vi "多参数全局变量.vi"() -> ()   [LabVIEW 2022 SP3, in "斯坦道原位多参数.lvlib"]
uses:
  <vilib>/Plasmionique/MB Master/MB_Master_Serial/MB_Master_Serial.lvclass
panel:
  in  "MB_Serial session in":refnum<class "MB_Master_Serial.lvclass">
  out "pHmv数据区":T1
  out "TDS数据区":T1
  out "spCond数据区":T1
  out "传感器通道号":T2
  out "Sal数据区":T1
  out "NH3N数据区":T1
  out "ORP数据区":T1
  out "蓝绿藻数据区":T1
  out "藻密度数据区":T1
  out "叶绿素数据区":T1
  out "Turb数据区":T1
  out "Cond数据区":T1
  out "DO%数据区":T1
  out "DO数据区":T1
  out "pH数据区":T1
  out "水温数据区":T1
  out "运行状态":string
  out "通讯状态":bool
  out "测量数据区":T3
  out "关键参数区":T4
  in  "控制命令":u16(ring) items=["启动测量"=1, "标样核查"=2, "零点核查"=3, "跨度核查"=4, "空白测试"=5, "平行样测试"=6, "加标回收"=7, "空白校准"=8, "标样校准"=9, "初始化（清洗）"=10, "停止测试"=11, "仪器重启"=12, "校时"=13, "模式设置"=14, "测量间隔设置"=15]
  out "状态告警区":T5
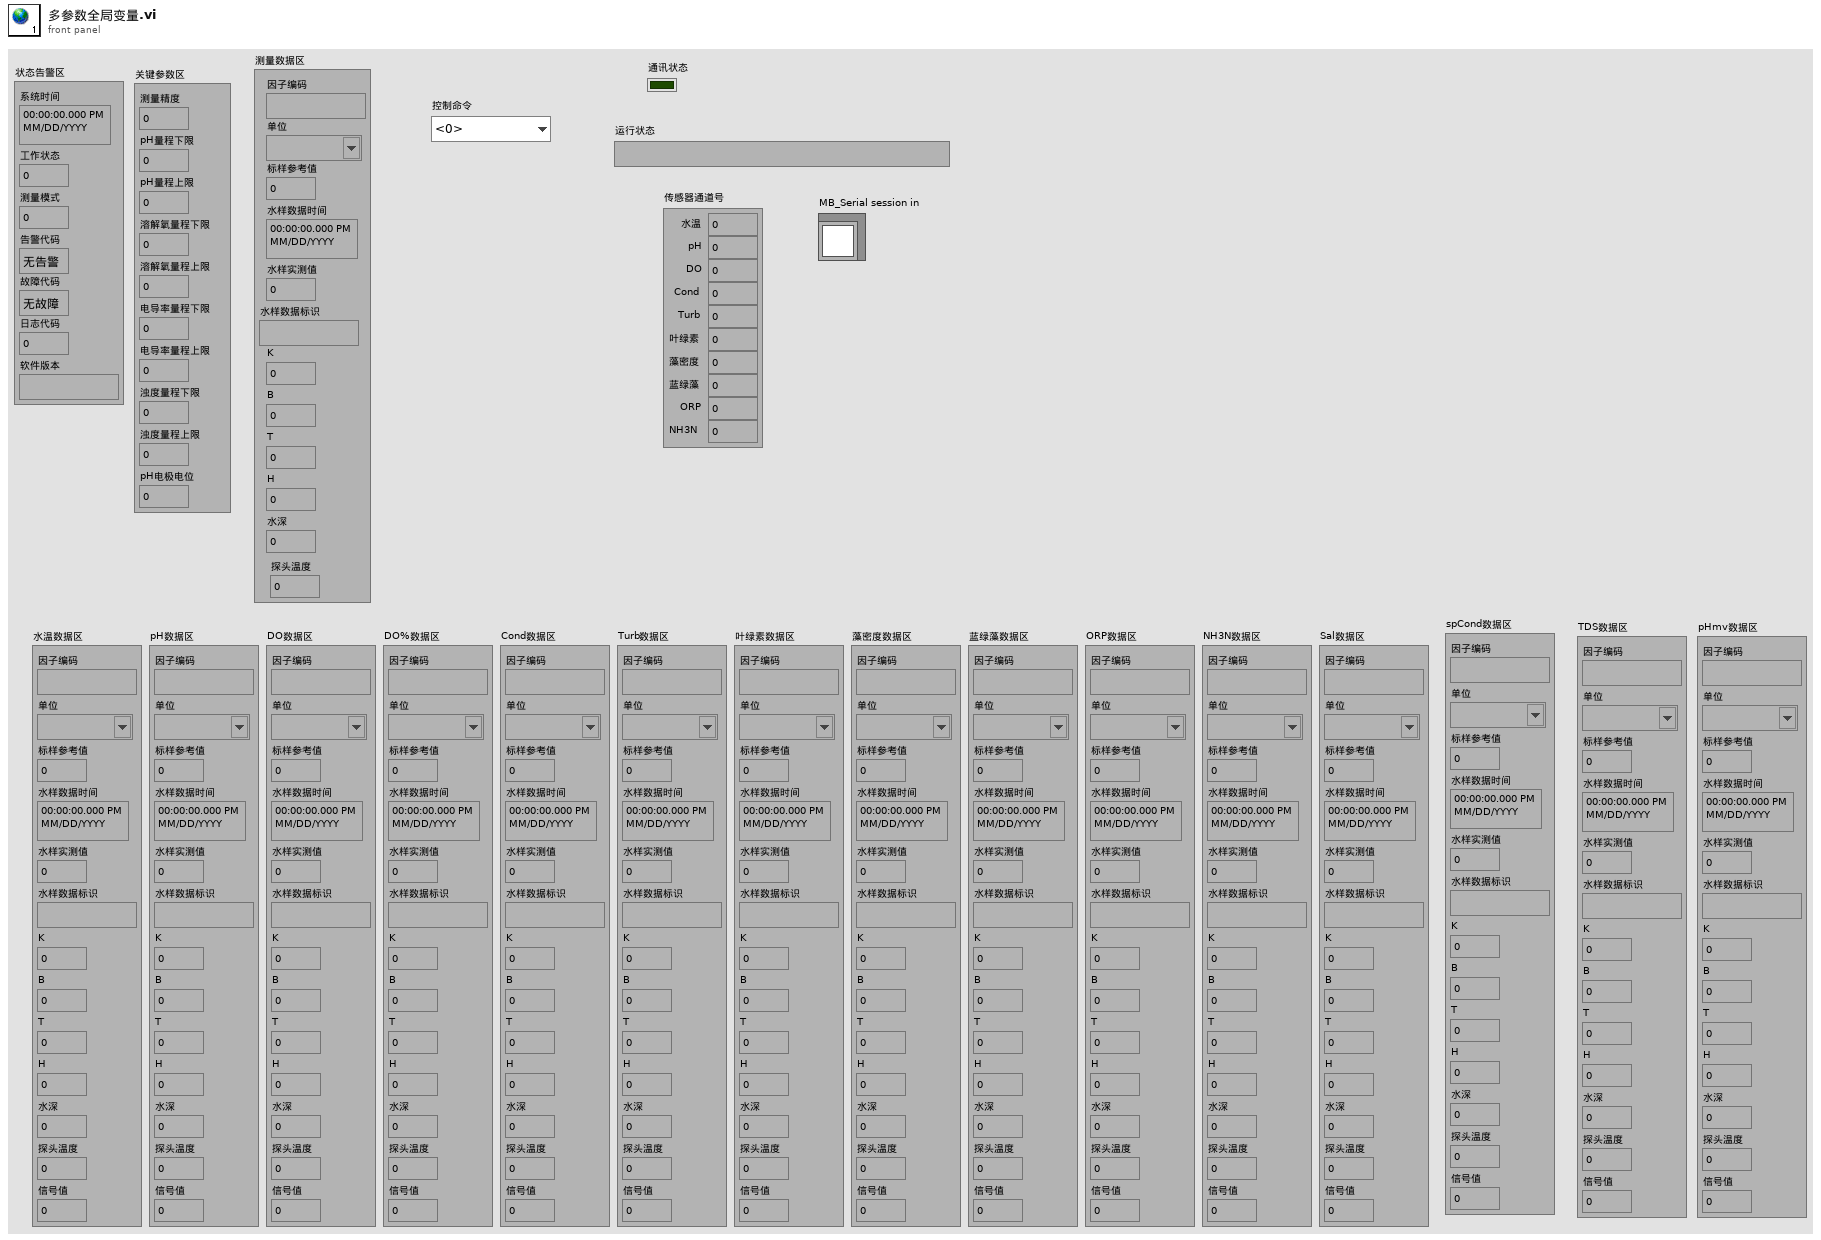
[diagram p1: front panel]
types:
  T1 = cluster{"因子编码":string, "单位":string, "标样参考值":sgl, "水样数据时间":timestamp, "水样实测值":sgl, "水样数据标识":string, "K":sgl, "B":sgl, "T":sgl, "H":sgl, "水深":sgl, "探头温度":sgl, "信号值":sgl}
  T2 = cluster{"水温":dbl, "pH":dbl, "DO":dbl, "Cond":dbl, "Turb":dbl, "叶绿素":dbl, "藻密度":dbl, "蓝绿藻":dbl, "ORP":dbl, "NH3N":dbl}
  T3 = cluster{"因子编码":string, "单位":string, "标样参考值":sgl, "水样数据时间":timestamp, "水样实测值":sgl, "水样数据标识":string, "K":sgl, "B":sgl, "T":sgl, "H":sgl, "水深":sgl, "探头温度":sgl}
  T4 = cluster{"测量精度":u16, "pH量程下限":sgl, "pH量程上限":sgl, "溶解氧量程下限":sgl, "溶解氧量程上限":sgl, "电导率量程下限":sgl, "电导率量程上限":sgl, "浊度量程下限":sgl, "浊度量程上限":sgl, "pH电极电位":sgl}
  T5 = cluster{"系统时间":timestamp, "工作状态":u16, "测量模式":u16, "告警代码":enum16{"无告警", "缺试剂告警", "缺水样告警", "缺蒸馏水告警", "缺标液告警", "仪表漏液告警", "标定异常告警", "超量程告警", "加热异常", "低试剂预警", "超上限告警", "超下限告警", "仪表内部其他异常", "滴定异常告警", "电极异常告警", "量程切换告警", "参数设置告警", "PH电极电位异常", "电导率电极异常", "浊度光度异常", "溶解氧电极异常", "溶解氧光强异常", "温度异常告警", "PH异常告警", "溶解氧异常告警", "电导率异常告警", "浊度异常告警", "叶绿素异常告警", "藻密度异常告警", "蓝绿藻异常告警", "ORP异常告警", "氨氮异常告警", "清洁刷异常告警", "SD卡异常告警", "蓝牙异常告警", "Wifi异常告警", "流程异常告警"}, "故障代码":enum16{"无故障", "电机故障", "温度故障", "通讯故障", "滴定故障"}, "日志代码":u16, "软件版本":string}
diagram:
